vi "TurnToAngleControllerSRX.vi"(0 "TargetAngle":dbl=600.0, 1 "MotionMagicTargets":cluster{"Pos":dbl, "Vel":dbl}={"Pos"=80.0, "Vel"=80.0}, 5 "Robot":T1={"Angle"=548.1299999999924, "Left Distance"=26.0882735, "Left vel"=0.0}, 9 "Gains":T2={"MinVoltage"=0.0, "Effective Trackwidth"=30.0}, 11 "Reset":bool, 13 "GoSmallestDistance":bool) -> (4 "TargetEncoderValue":dbl, 6 "MinVoltage":dbl, 8 "Encoder Distance":cluster{"Output":dbl, "dx/dt":dbl}(graph)={"Output"=52.36486996421861, "dx/dt"=26.0882735}, 12 "Angle":cluster{"Distance":dbl, "CurrentAngle":dbl}(graph)={"Distance"=-120.0, "CurrentAngle"=-171.87000000000762}, 14 "VelGraph":cluster{"Output":dbl, "dx/dt":dbl}(graph), 15 "Done":bool)   [LabVIEW 2018]
panel:
  in  "Target Vel":dbl
  out "Delay":dbl=20.0
  in  "MaxAccel":dbl=150.0
  in  "MaxVel":dbl=80.0
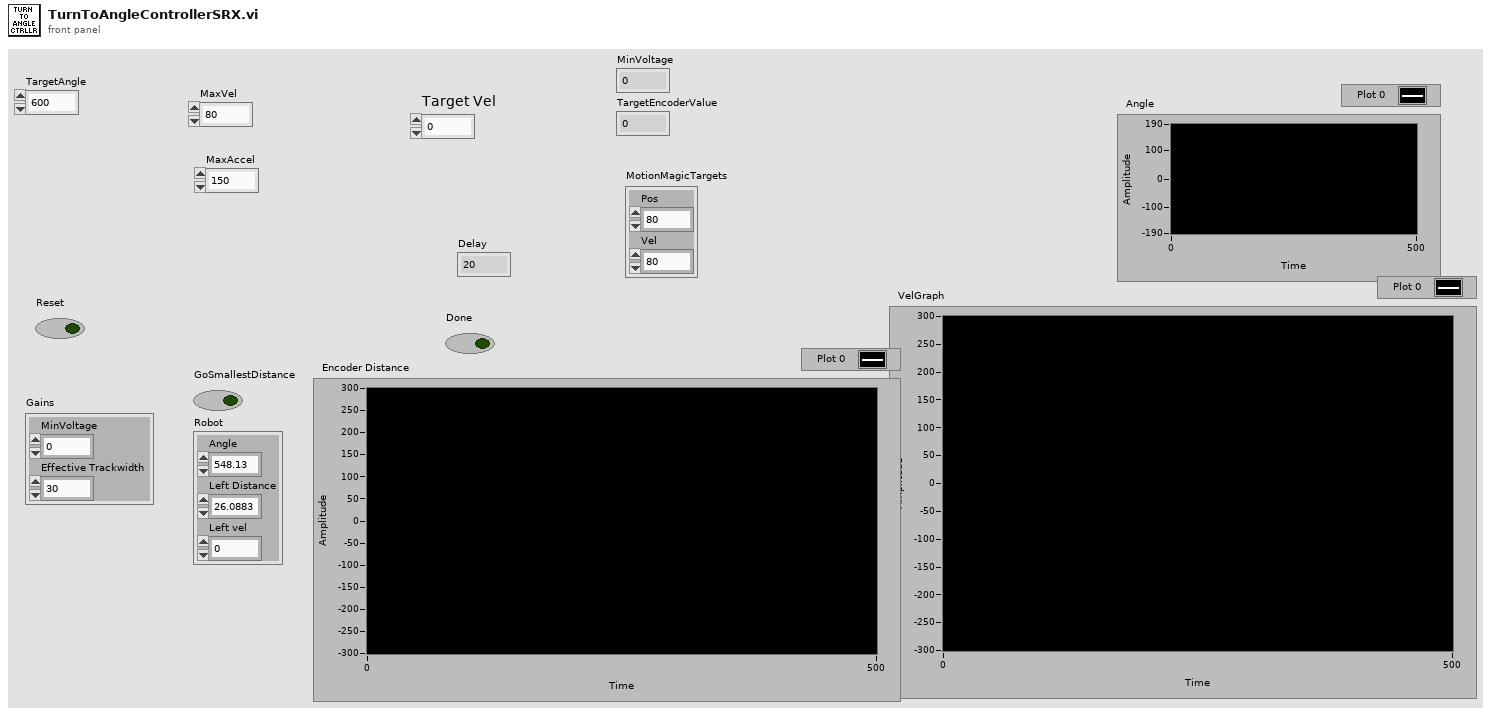
[diagram p1: front panel]
types:
  T1 = cluster{"Angle":dbl, "Left Distance":dbl, "Left vel":dbl}
  T2 = cluster{"MinVoltage":dbl, "Effective Trackwidth":dbl}
  T3 = cluster{"Smallest A to B":dbl, "Smallest A to B":dbl}
  T4 = cluster{"Smallest A to B":dbl, "Left Distance":dbl}
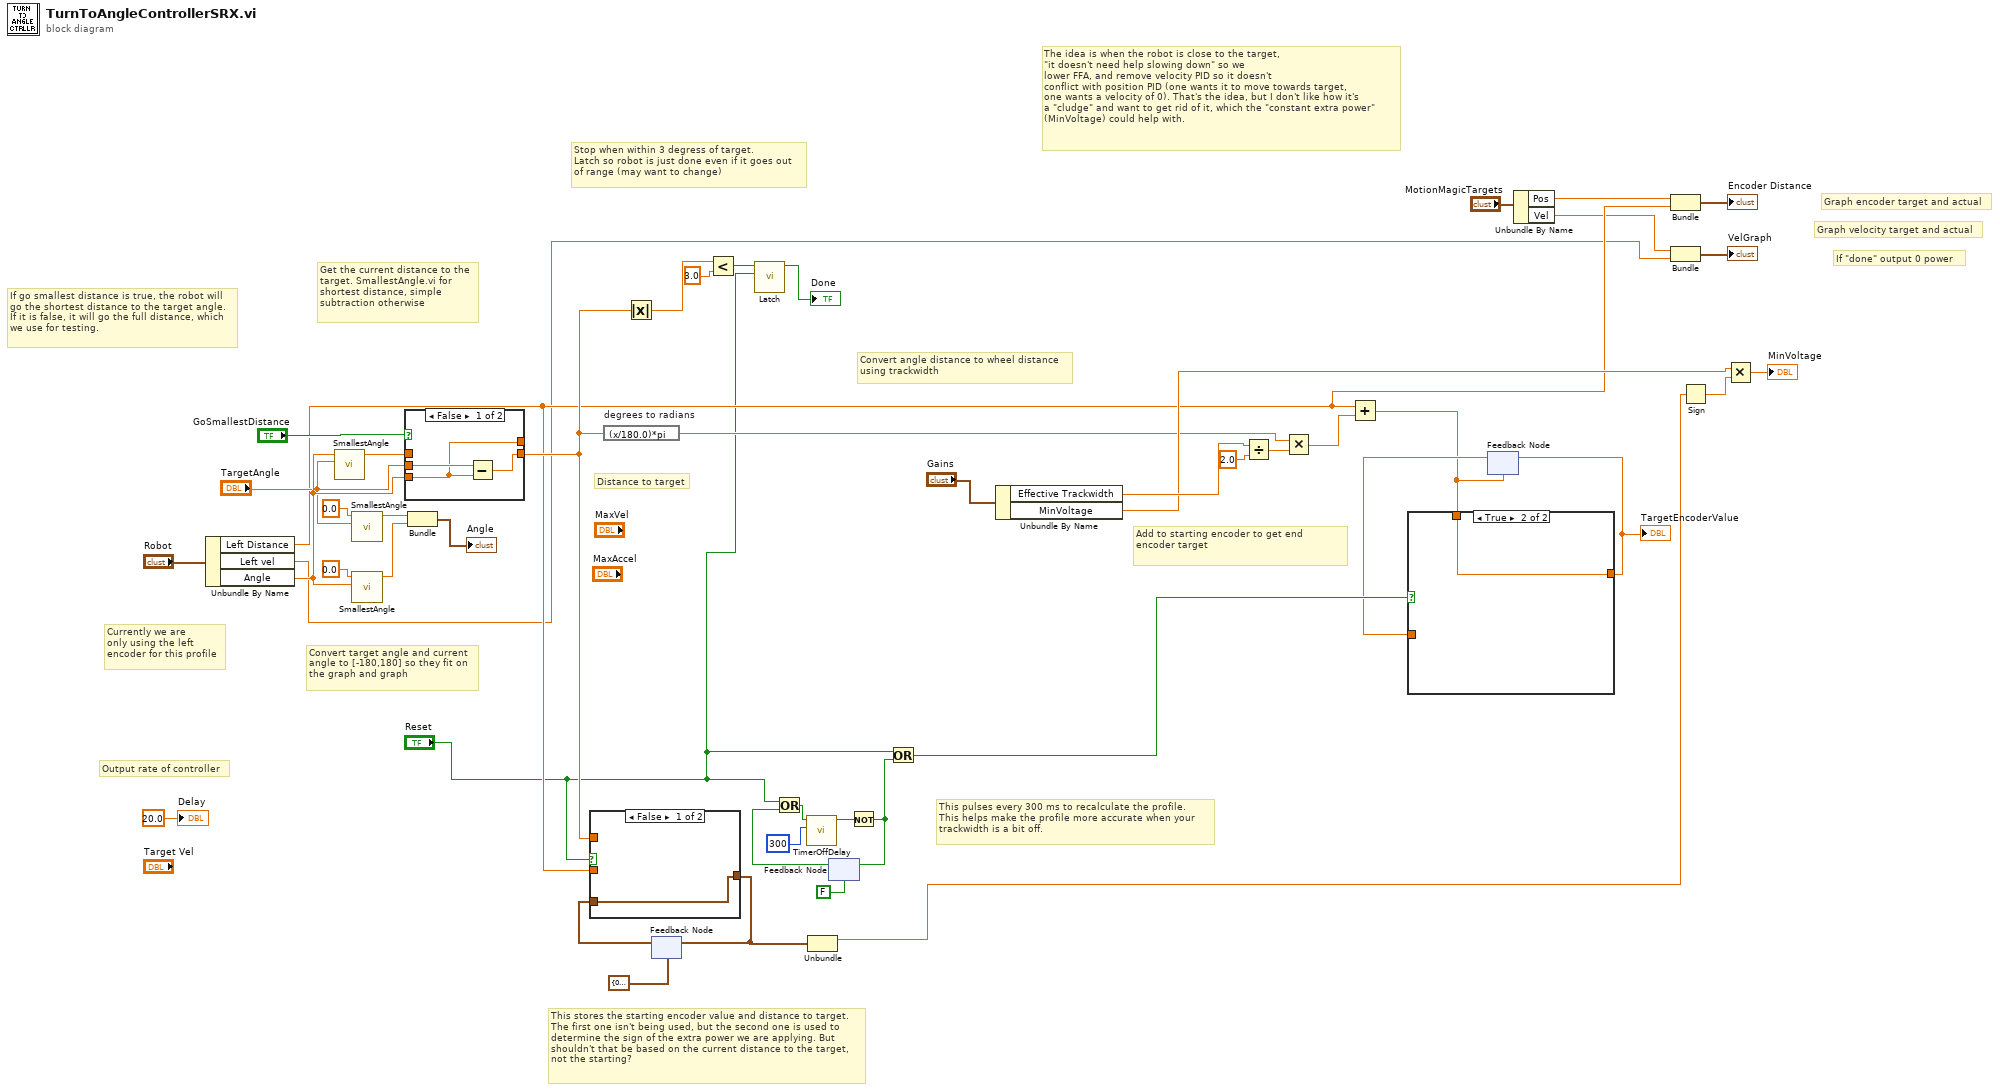
[diagram p0: block diagram]
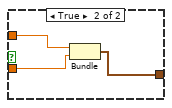
[diagram p3: hidden frame]
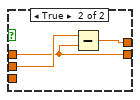
[diagram p4: hidden frame]
diagram:
  # "Currently we are\nonly using the left\nencoder for this profile"
  # "Output rate of controller"
  # "If \"done\" output 0 power"
  # "Graph velocity target and actual"
  # "Graph encoder target and actual"
  # "The idea is when the robot is close to the target,\n\"it doesn't need help slowing down\" so we\nlower FFA, and remove velocity PID so it doesn't\nconflict with position PID (one wants it to move towards target,\none wants a velocity of 0). That's the idea, but I don't like how it's\na \"cludge\" and want to get rid of it, which the \"constant extra power\"\n(MinVoltage) could help with."
  # "Add to starting encoder to get end\nencoder target"
  # "Convert angle distance to wheel distance\nusing trackwidth"
  # "This pulses every 300 ms to recalculate the profile.\nThis helps make the profile more accurate when your\ntrackwidth is a bit off."
  # "This stores the starting encoder value and distance to target.\nThe first one isn't being used, but the second one is used to\ndetermine the sign of the extra power we are applying. But\nshouldn't that be based on the current distance to the target,\nnot the starting?"
  # "Stop when within 3 degress of target.\nLatch so robot is just done even if it goes out\nof range (may want to change)"
  # "Get the current distance to the\ntarget. SmallestAngle.vi for \nshortest distance, simple\nsubtraction otherwise"
  # "If go smallest distance is true, the robot will\ngo the shortest distance to the target angle.\nIf it is false, it will go the full distance, which\nwe use for testing."
  # "Convert target angle and current\nangle to [-180,180] so they fit on\nthe graph and graph"
  # "Distance to target"
  n1 = Unbundle By Name("Robot") -> ("Left Distance"=w22:dbl, "Left vel"=w12:dbl, "Angle"=w38:dbl)
  n2 = call "SmallestAngle.vi"("Angle B"="TargetAngle", "Angle A"=w38) -> ("Smallest A to B"=w44:dbl)  [unwired: 9 in]
  n3 = call "SmallestAngle.vi"("Angle B"="TargetAngle", "Angle A"=0.0) -> ("Smallest A to B"=w36:dbl)  [unwired: 9 in]
  n4 = call "SmallestAngle.vi"("Angle B"=w38, "Angle A"=0.0) -> ("Smallest A to B"=w35:dbl)  [unwired: 9 in]
  n5 = case shown="False" "GoSmallestDistance" {
    tunnel: [w49 w53] -> _
    tunnel: "TargetAngle" -> [w50 w52]
    tunnel: w44 -> [_ w51]
    tunnel: [w48 w51] -> w23
    tunnel: w38 -> [w49 _]
    frame False {
      n6 = Subtract(x=w50, y=w49) -> (x-y=w48:dbl)
    }
    frame True {
      n7 = Subtract(x=w52, y=w51) -> (x-y=w53:dbl)
    }
  }
  n8 = Bundle("Smallest A to B"=w36, "Smallest A to B"=w35) -> (→"Angle":T3)  [unwired: 1 in]
  n9 = expression code="(x/180.0)*pi" "degrees to radians"(w23) -> (w21:dbl)
  n10 = Absolute Value(x=w23) -> (abs(x)=w28:dbl)
  n11 = feedback #1(cluster{"Angle":dbl, "Distance":dbl} {"Angle"=0.0, "Distance"=0.0}) -> (w30:cluster{"Angle":dbl, "Distance":dbl})
  n12 = case shown="False" "Reset" {
    tunnel: w23 -> [_ w57]
    tunnel: [w54 w56] -> w20
    tunnel: w30 -> [w54 _]
    tunnel: w22 -> [_ w55]
    frame False {
    }
    frame True {
      n13 = Bundle("Smallest A to B"=w57, "Left Distance"=w55) -> (w56:T4)  [unwired: 1 in]
    }
  }
  n14 = feedback-in #1(w20) -> ()
  n15 = Less?(x=w28, y=3.0) -> (x < y?=w42:bool)
  n16 = call "Latch.vi"("Reset"="Reset", "Input"=w42) -> ("Output"=→"Done":bool)  [unwired: 9 in]
  n17 = Unbundle(w20) -> ("Smallest A to B"=w19:dbl)  [unwired: 1 out]
  n18 = feedback #2(FALSE) -> (w15:bool)
  n19 = Or(x="Reset", y=w15) -> (x .or. y?=w16:bool)
  n20 = call "TimerOffDelay.vi"("Time Delay"=u32 300, "Input"=w16) -> ("Output"=w14:bool)  [unwired: 9 in]
  n21 = Not(x=w14) -> (.not. x?=w13:bool)
  n22 = feedback-in #2(w13) -> ()
  n23 = Or(x="Reset", y=w13) -> (x .or. y?=w9:bool)
  n24 = Unbundle By Name("Gains") -> ("Effective Trackwidth"=w29:dbl, "MinVoltage"=w26:dbl)
  n25 = Divide(x=w29, y=2.0) -> (x/y=w33:dbl)
  n26 = Multiply(x=w21, y=w33) -> (x*y=w32:dbl)
  n27 = Add(x=w22, y=w32) -> (x+y=w6:dbl)
  n28 = feedback #3(w6) -> (w7:dbl)
  n29 = case shown="True" w9 {
    tunnel: [w58 w59] -> w8
    tunnel: w6 -> [_ w59]
    tunnel: w7 -> [w58 _]
    frame False {
    }
    frame True {
    }
  }
  "TargetEncoderValue" <- w8
  n30 = feedback-in #3(w8) -> ()
  n31 = Unbundle By Name("MotionMagicTargets") -> ("Pos"=w4:dbl, "Vel"=w3:dbl)
  n32 = Bundle("Pos"=w4, "Left Distance"=w22) -> (→"Encoder Distance":cluster{"Pos":dbl, "Left Distance":dbl})  [unwired: 1 in]
  n33 = Bundle("Vel"=w3, "Left vel"=w12) -> (→"VelGraph":cluster{"Vel":dbl, "Left vel":dbl})  [unwired: 1 in]
  n34 = Sign(1:w19) -> (0:w27:dbl)
  n35 = Multiply(x=w26, y=w27) -> (x*y=→"MinVoltage":dbl)
  "Delay" <- 20.0 ("Time Left")
